vi "切换界面.vi"(8 "error in (no error)":errorcluster caption="错误输入（无错误）", 9 "界面":bool, 10 "布尔控件":refnum<vi>, 11 "程序响应 输入":refnum<class "程序响应.lvclass">) -> (0 "error out":errorcluster caption="错误输出", 3 "程序响应 输出":refnum<class "程序响应.lvclass">)   [LabVIEW 2020, in "程序响应.lvlib" / "程序响应.lvclass"]
uses:
  D:/SuperPython-master/ScintillaNET.dll
  ScintillaNET.dll
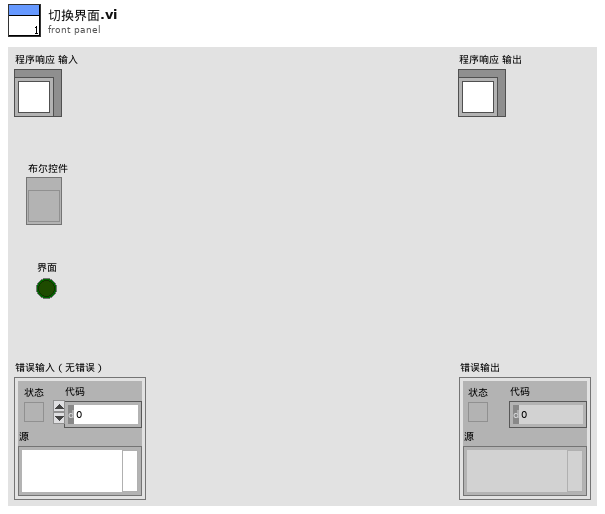
[diagram p1: front panel]
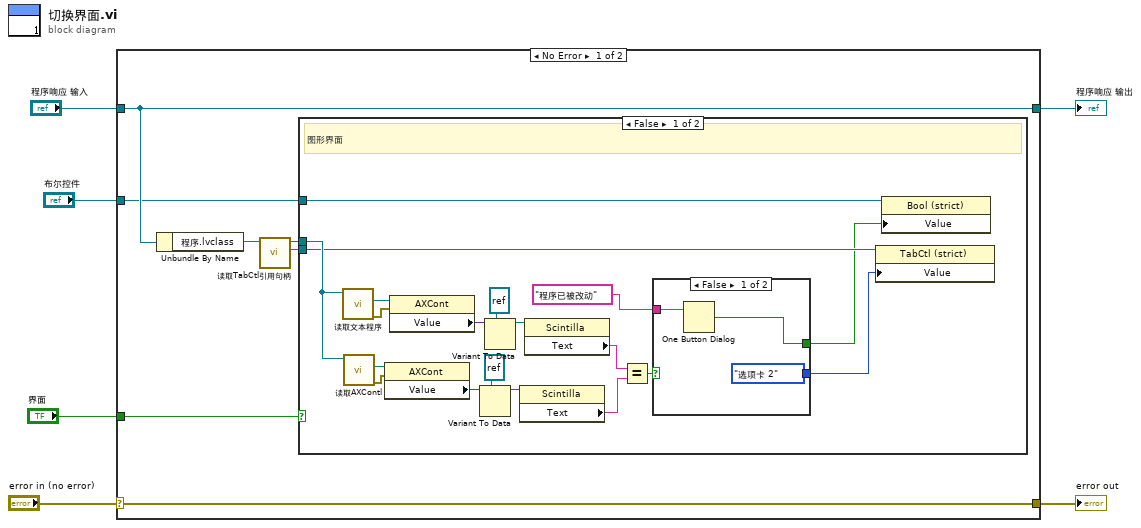
[diagram p0: block diagram]
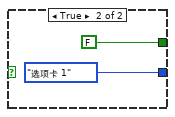
[diagram p2: hidden frame]
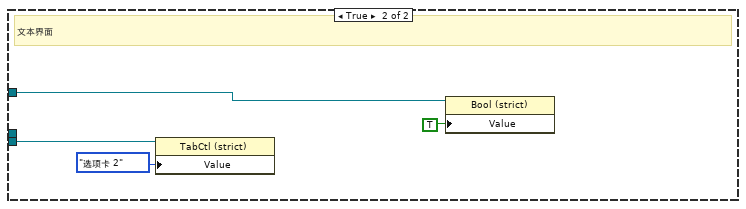
[diagram p3: hidden frame]
diagram:
  n1 = case shown="No Error" "error in (no error)" {
    selector: "error in (no error)" -> [w13 w43]
    tunnel: [w13 w43] -> w5
    tunnel: [w12 w42] -> w3
    tunnel: "程序响应 输入" -> [w12 w42]
    tunnel: "界面" -> [w11 _]
    tunnel: "布尔控件" -> [w7 _]
    frame No Error {
      n2 = Unbundle By Name(w12) -> ("程序.lvclass"=w9:refnum<class "程序.lvclass">)
      n3 = call-dynamic "读取TabCtl引用句柄.vi"("程序输入"=w9) -> ("TabCtl引用句柄"=w10:refnum<vi>, "程序输出"=w8:refnum<class "程序.lvclass">)  [unwired: 8 in, 1 out]
      n4 = case shown="False" w11 {
        tunnel: w8 -> [w32 _]
        tunnel: w10 -> [w19 w41]
        tunnel: w7 -> [w16 w39]
        frame False {
          # "图形界面"
          n5 = call-dynamic "读取文本程序.vi"("程序输入"=w32) -> ("error out"=w24:errorcluster, "文本程序"=w29:refnum<vi>)  [unwired: 8 in, 1 out]
          n6 = call-dynamic "读取AXContl.vi"("程序输入"=w32) -> ("error out"=w25:errorcluster, "AXContl"=w26:refnum<vi>)  [unwired: 8 in, 1 out]
          n7 = property class="AXCont"(reference=w26, error in=w25) -> ("Value"=w28:variant)  [unwired: 2 out]
          n8 = property class="AXCont"(reference=w29, error in=w24) -> ("Value"=w30:variant)  [unwired: 2 out]
          n9 = Variant To Data(type=refnum<k24> refnum ("文本编辑"), Variant=w28) -> (data=w27:refnum<k24>)  [unwired: 1 in, 1 out]
          n10 = Variant To Data(type=refnum<k24> refnum ("文本编辑"), Variant=w30) -> (data=w31:refnum<k24>)  [unwired: 1 in, 1 out]
          n11 = property class="Scintilla"(reference=w27) -> ("Text"=w20:string)  [unwired: 1 in, 2 out]
          n12 = property class="Scintilla"(reference=w31) -> ("Text"=w21:string)  [unwired: 1 in, 2 out]
          n13 = Equal?(x=w21, y=w20) -> (x = y?=w18:bool)
          n14 = case shown="False" w18 {
            tunnel: [enum32{"选项卡 1", "选项卡 2"}."选项卡 2" ("值") enum32{"选项卡 1", "选项卡 2"}."选项卡 1" ("值")] -> w17
            tunnel: [w33 FALSE] -> w15
            tunnel: "程序已被改动" -> [w34 _]
            frame False {
              n15 = One Button Dialog(message=w34) -> (true=w33:bool)  [unwired: 1 in]
            }
            frame True {
            }
          }
          n16 = property class="TabCtl (strict)"(reference=w19, "Value"=w17) -> ()  [unwired: 1 in, 2 out]
          n17 = property class="Bool (strict)"(reference=w16, "Value"=w15) -> ()  [unwired: 1 in, 2 out]
        }
        frame True {
          # "文本界面"
          n18 = property class="TabCtl (strict)"(reference=w41, "Value"=enum32{"选项卡 1", "选项卡 2"}."选项卡 2" ("值")) -> ()  [unwired: 1 in, 2 out]
          n19 = property class="Bool (strict)"(reference=w39, "Value"=TRUE ("值")) -> ()  [unwired: 1 in, 2 out]
        }
      }
    }
    frame Error {
    }
  }
  "error out" <- w5
  "程序响应 输出" <- w3
